vi "init_fw103h.vi"(8 "SerialNumber":string="40154488") -> (0 "Initialised":bool=TRUE, 1 "Method reference":refnum<k24>, 2 "Device reference":refnum<k24>, 3 "error out":errorcluster)   [LabVIEW 2020]
uses:
  C:/Users/OPMuser/Documents/labview/fw103/Thorlabs.MotionControl.Controls.dll
  Thorlabs.MotionControl.Controls.dll
  C:/Users/OPMuser/Documents/labview/fw103/Thorlabs.MotionControl.Benchtop.StepperMotorCLI.dll
  Thorlabs.MotionControl.Benchtop.StepperMotorCLI.dll
panel:
  in  "BenchtopStepperControl":refnum<k24>(container)
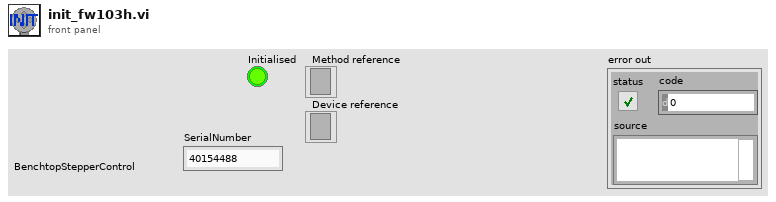
[diagram p1: front panel]
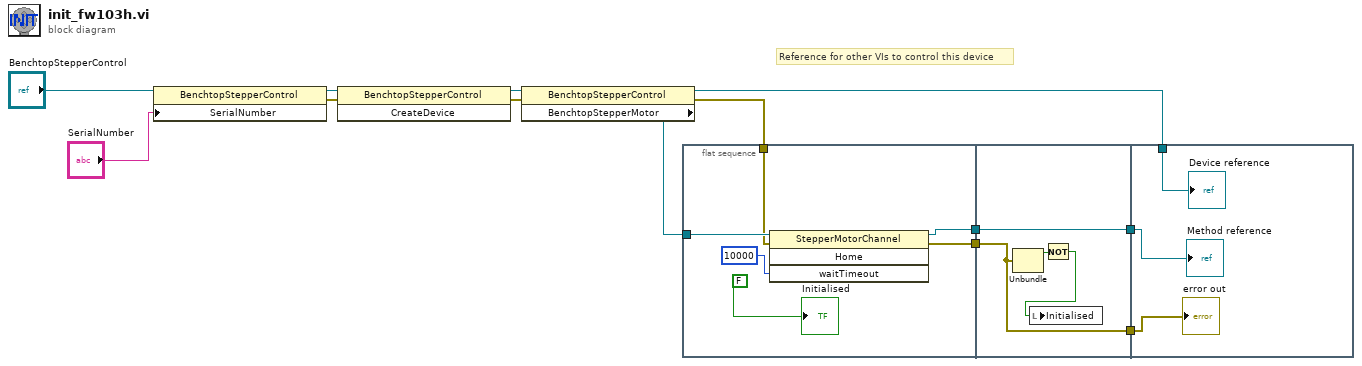
[diagram p0: block diagram]
diagram:
  # "Reference for other VIs to control this device"
  n1 = property class="BenchtopStepperControl"(reference="BenchtopStepperControl", "SerialNumber"="SerialNumber") -> (reference out=w11:refnum<k24>, error out=w7:errorcluster)  [unwired: 1 in]
  n2 = invoke class="BenchtopStepperControl" method="CreateDevice"(reference=w11, error in=w7) -> (reference out=w10:refnum<k24>, error out=w6:errorcluster)  [unwired: 1 in, 1 out]
  n3 = property class="BenchtopStepperControl"(reference=w10, error in=w6) -> (reference out=w1:refnum<k24>, error out=w5:errorcluster, "BenchtopStepperMotor"=w9:refnum<k24>)
  n4 = flat-sequence {
    tunnel: w9 -> [w19]
    tunnel: [w17] -> w8
    tunnel: w5 -> [w16]
    tunnel: [w15] -> w4
    tunnel: w8 -> [w23]
    tunnel: w4 -> [w20]
    tunnel: [w23] -> w3
    tunnel: [w20] -> w2
    tunnel: w3 -> [w25]
    tunnel: w2 -> [w26]
    tunnel: w1 -> [w24]
    frame #0 {
      n5 = invoke class="StepperMotorChannel" method="Home"(reference=w19, error in=w16, "waitTimeout"=10000) -> (reference out=w17:refnum<k24>, error out=w15:errorcluster)  [unwired: 1 in, 2 out]
      "Initialised" <- FALSE ("Initialised")
    }
    frame #1 {
      n6 = Unbundle(w20) -> ("status"=w22:bool)  [unwired: 2 out]
      n7 = Not(x=w22) -> (.not. x?=w21:bool)
      n8 = local write "Initialised"(w21) -> ()
    }
    frame #2 {
      "Method reference" <- w25
      "error out" <- w26
      "Device reference" <- w24
    }
  }
